vi "append.vi"(8 "error in (no error)":errorcluster, 9 "data":dbl[](array[numeric]) format="%0.2f", 10 "current time":timestamp, 11 "data log in":refnum<class "data log.lvclass">) -> (0 "error out":errorcluster, 3 "data log out":refnum<class "data log.lvclass">)   [LabVIEW 2025, in "data log.lvclass"]
uses:
  data log.lvclass
  data log.lvclass/data log.ctl
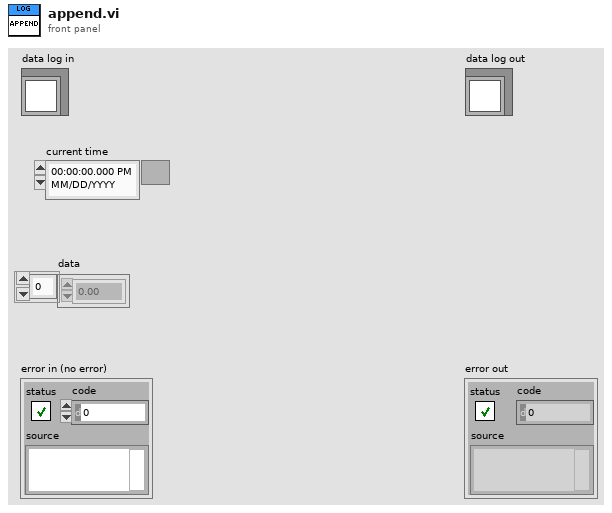
[diagram p1: front panel]
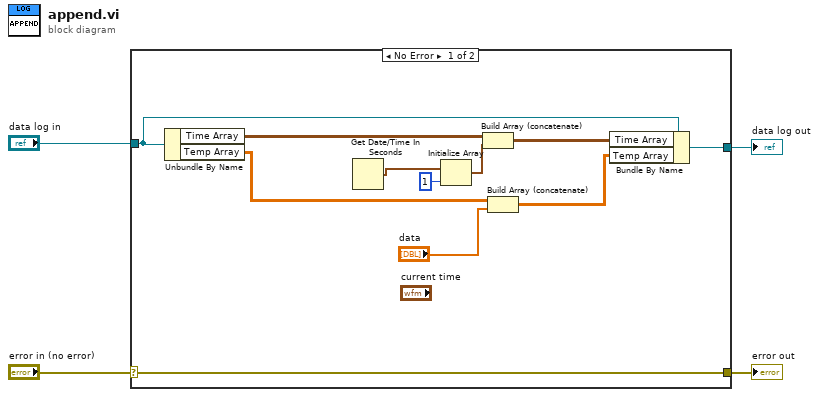
[diagram p0: block diagram]
diagram:
  n1 = case shown="No Error" "error in (no error)" {
    selector: "error in (no error)" -> [w15 w17]
    tunnel: [w15 w17] -> w3
    tunnel: [w11 w16] -> w1
    tunnel: "data log in" -> [w10 w16]
    frame No Error {
      n2 = Unbundle By Name(w10) -> ("Time Array"=w13:timestamp[][], "Temp Array"=w12:dbl[][])
      n3 = Get Date/Time In Seconds() -> (seconds since 1Jan1904=w7:timestamp)
      n4 = Initialize Array(w7, 1 ("dimension size")) -> (w5:timestamp[])
      n5 = Build Array (concatenate)(w13, w5) -> (w9:timestamp[][])
      n6 = Build Array (concatenate)(w12, "data") -> (w8:dbl[][])
      n7 = Bundle By Name(cluster=w10, "Time Array"=w9, "Temp Array"=w8) -> (w11:refnum<class "data log.lvclass">)
    }
    frame Error {
    }
  }
  "error out" <- w3
  "data log out" <- w1
